vi "Read (Multiple Points).vi"(8 "error in (no error)":errorcluster, 9 "Timeout (10000 ms)":i32=10000, 10 "Sample Count (1)":i32=1, 11 "VISA resource name":refnum<visa-resource-name>) -> (0 "error out":errorcluster, 2 "Measurements":dbl[](array[numeric]), 3 "VISA resource name out":refnum<visa-resource-name>)   [LabVIEW 2014, in "Fluke 884X Series.lvlib"]
doc: "Reads and returns multiple measurements from the instrument. Use this VI when you want to take multiple measurements using an immediate trigger. Use the low level VIs for other triggering options."
uses:
  Fluke 884X Series.lvlib
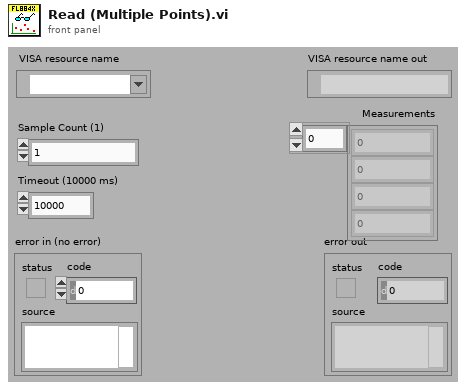
[diagram p1: front panel]
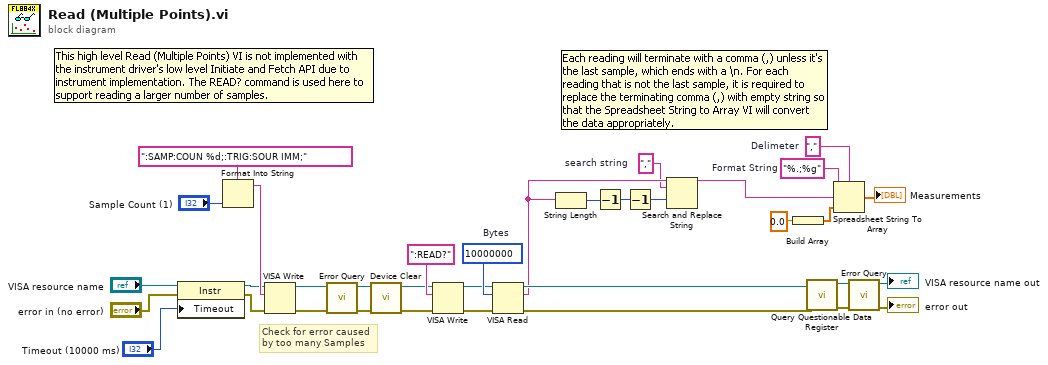
[diagram p0: block diagram]
diagram:
  w1 = ","  # search string
  w27 = ","  # Delimeter
  w28 = "%.;%g"  # Format String
  w29 = u32 10000000  # Bytes
  # "Check for error caused by too many Samples"
  n1 = property on="Property Node" class="Instr"(reference="VISA resource name", error in="error in (no error)", "Timeout"="Timeout (10000 ms)") -> (reference out=w16:refnum<visa-resource-name>, error out=w15:errorcluster)
  n2 = Format Into String(format string=":SAMP:COUN %d;:TRIG:SOUR IMM;" ("Sample Count"), "Sample Count (1)") -> (resulting string=w31:string)  [unwired: 2 in, 1 out]
  n3 = VISA Write(VISA resource name=w16, write buffer=w31, error in (no error)=w15) -> (VISA resource name out=w20:refnum<visa-resource-name>, error out=w21:errorcluster)  [unwired: 1 out]
  n4 = call "Error Query.vi"("error in (no error)"=w21, "VISA resource name"=w20) -> ("error out"=w13:errorcluster, "VISA resource name out"=w14:refnum<visa-resource-name>)  [unwired: 6 in, 2 out]
  n5 = call "Device Clear.vi"("error in (no error)"=w13, "VISA Resource Name"=w14) -> ("error out"=w11:errorcluster, "VISA Resource Out"=w12:refnum<visa-resource-name>)  [unwired: 8 in]
  n6 = VISA Write(VISA resource name=w12, write buffer=":READ?" ("Read Measurement"), error in (no error)=w11) -> (VISA resource name out=w10:refnum<visa-resource-name>, error out=w9:errorcluster)  [unwired: 1 out]
  n7 = VISA Read(VISA resource name=w10, byte count=w29, error in (no error)=w9) -> (VISA resource name out=w5:refnum<visa-resource-name>, read buffer=w3:string, error out=w4:errorcluster)  [unwired: 1 out]
  n8 = String Length(string=w3) -> (length=w6:i32)
  n9 = Decrement(x=w6) -> (x-1=w7:i32)
  n10 = Decrement(x=w7) -> (x-1=w8:i32)
  n11 = Search and Replace String(input string=w3, search string=w1, offset=w8) -> (result string=w2:string)  [unwired: 5 in, 3 out]
  n12 = Build Array(0.0) -> (w25:dbl[])
  n13 = call "Query Questionable Data Register.vi"("error in (no error)"=w4, "VISA resource name"=w5) -> ("error out"=w22:errorcluster, "VISA resource name out"=w23:refnum<visa-resource-name>)  [unwired: 7 in, 1 out]
  n14 = Spreadsheet String To Array(delimiter (Tab)=w27, format string=w28, spreadsheet string=w2, array type (2D Dbl)=w25) -> (array=→"Measurements":dbl[])
  n15 = call "Error Query.vi"("error in (no error)"=w22, "VISA resource name"=w23) -> ("error out"=→"error out":errorcluster, "VISA resource name out"=→"VISA resource name out":refnum<visa-resource-name>)  [unwired: 6 in, 2 out]
